vi "SetSizeAndOriginForMultiplot.vi"(4 "VerticalPosition":dbl, 5 "Height":dbl, 6 "LateralPosition":dbl, 7 "Width":dbl, 9 "PlotLocationDescription":string="Top-left plot", 11 "gnuplotIn":string) -> (3 "gnuplotOut":string)   [LabVIEW 2013]
panel:
  out "resulting string":string
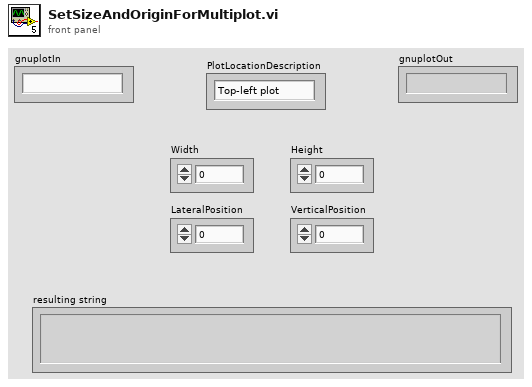
[diagram p1: front panel]
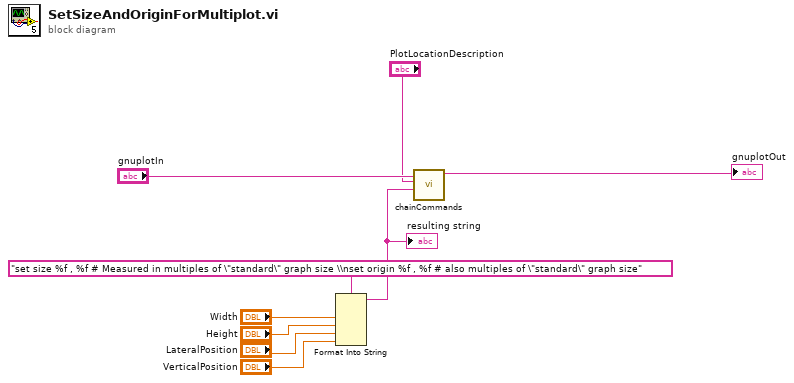
[diagram p0: block diagram]
diagram:
  n1 = Format Into String(format string="set size %f , %f # Measured in multiples of \"standard\" graph size \\nset origin %f , %f # also multiples of \"standard\" graph size", "Width", "Height", "LateralPosition", "VerticalPosition") -> (resulting string=w1:string)  [unwired: 2 in, 1 out]
  "resulting string" <- w1
  n2 = call "chainCommands.vi"("Command"=w1, "Comments"="PlotLocationDescription", "StringIn"="gnuplotIn") -> ("StringOut"=→"gnuplotOut":string)  [unwired: 8 in]
